vi "fix_issue_dates.vi"(7 "root paths":cluster{"cv_volumes":path, "cv_issues":path}={"cv_volumes"=path "D:/Comics/data/cv_volumes", "cv_issues"=path "D:/Comics/data/cv_issues"}, 8 "error in (no error)":errorcluster, 10 "volume":string, 11 "manager_daemon in":refnum<class "manager_daemon.lvclass">) -> (0 "error out":errorcluster)   [LabVIEW 2024]
uses:
  comic_manager/manager_daemon/manager_daemon.lvclass
  CV_Shared_Library/CV_Shared_Library.lvlib
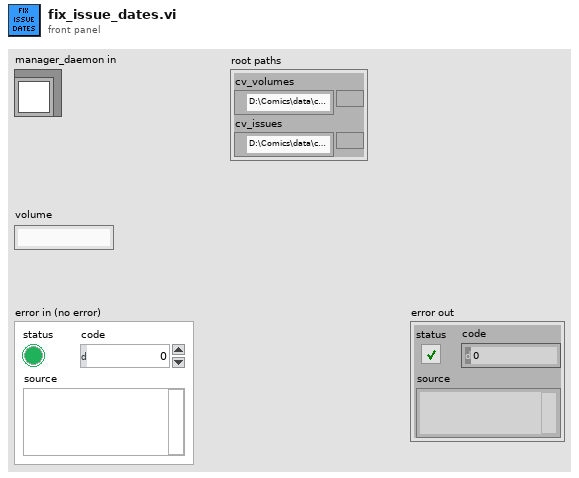
[diagram p1: front panel]
types:
  T1 = typedef "CV_RESTful_Lib.lvlib/local_volume--cluster.ctl" = cluster{"id":i32, "name":string, "sortable_name":string, "aliases":string[], "description":string, "site_detail_url":string, "count_of_issues":i32, "start_year":i32, "publisher_id":i32, "issue_ids":i32[], "date_last_updated":timestamp, "volume":i32, "cv_id":string, "volume type":T2}
  T2 = typedef "CV_Shared_Library.lvlib/volume.type--enum.ctl" = enum16{"Ongoing", "Limited Series", "Annual", "One Shot", "Reprint/Document", "Star Comics", "Epic Comics"}
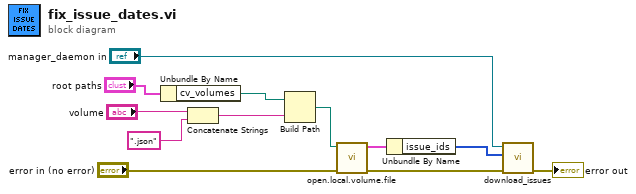
[diagram p0: block diagram]
diagram:
  n1 = Unbundle By Name("root paths") -> ("cv_volumes"=w9:path)
  n2 = Concatenate Strings("volume", ".json" ("string")) -> (w8:string)
  n3 = Build Path(base path=w9, name or relative path=w8) -> (appended path=w7:path)
  n4 = call "open.local.volume.file.vi"("error in (no error)"="error in (no error)", "volume json"=w7) -> ("error out"=w1:errorcluster, "volume"=w5:T1)  [unwired: 8 in]
  n5 = Unbundle By Name(w5) -> ("issue_ids"=w2:i32[])
  n6 = call "download_issues.vi"("error in (no error)"=w1, "issue ids"=w2, "manager_daemon in"="manager_daemon in") -> ("error out"=→"error out":errorcluster)  [unwired: 7 in, 1 out]
